vi "Format Numeric Tag.vi"(8 "Number":i32, 11 "Tree label":string) -> (3 "Tag":string)   [LabVIEW 2020, in "Output Sequencer.lvlib" / "Settings UI.lvclass"]
uses:
  Settings UI.lvclass
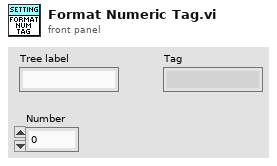
[diagram p1: front panel]
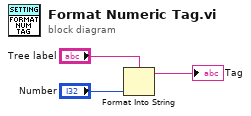
[diagram p0: block diagram]
diagram:
  n1 = Format Into String(format string="Tree label", "Number") -> (resulting string=→"Tag":string)  [unwired: 2 in, 1 out]
